vi "vms_getEvent_ErrorCode.vi"(8 "error in (no error)":errorcluster, 11 "logevent_ErrorCode_Ctl":T1) -> (0 "error out":errorcluster, 2 "function return":i32, 3 "logevent_ErrorCode_Ctl out":T1)   [LabVIEW 2016, in "SALLV_vms.lvlib"]
doc: "int vms_shm_getEvent_ErrorCodeLV(vms_logevent_ErrorCodeLV *logevent_ErrorCode_Ctl );"
uses:
  SALLV_vms.lvlib
  DataTypes/logevent_ErrorCode.ctl
  SALLV_vms.so
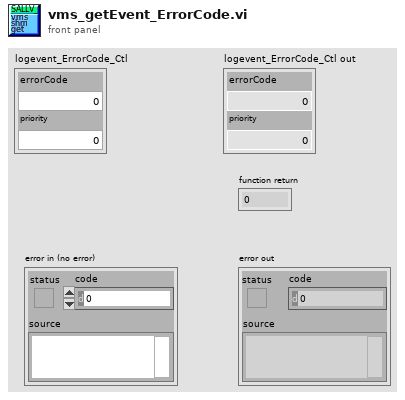
[diagram p1: front panel]
types:
  T1 = typedef "SALLV_vms.lvlib/logevent_ErrorCode.ctl" = cluster{"errorCode":i32, "priority":i32}
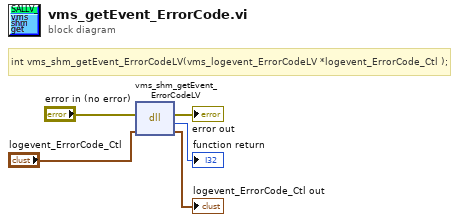
[diagram p0: block diagram]
diagram:
  # "int vms_shm_getEvent_ErrorCodeLV(vms_logevent_ErrorCodeLV *logevent_ErrorCode_Ctl );"
  n1 = dll-call lib="opt/CODE/SALLV_vms/SALLV_vms.*" fn="vms_shm_getEvent_ErrorCodeLV"(error in="error in (no error)", "logevent_ErrorCode_Ctl"="logevent_ErrorCode_Ctl") -> (error out=→"error out":errorcluster, →"function return":i32, "logevent_ErrorCode_Ctl"=→"logevent_ErrorCode_Ctl out":T1)  [unwired: 2 in, 1 out]
